vi "Enque Block (SubVI).vi"(10 "Block Parameters":T1={"Pixels In"=0, "BBox Array"=[0, 0, 0, 0, 0, 0, 0, 0, 0, 0, 0, 0, 0, 0, 0, 0], "Image Height"=0, "Image Width"=0, "Input Valid?"=FALSE, "Pixel Bus"={"Pixel Valid"=FALSE, "EOL"=FALSE, "EOF"=FALSE, "X"=0, "Y"=0}}, 11 "BOX ID":i32) -> (1 "Pixel Valid?":bool, 3 "Pixel Data":u8)   [LabVIEW 2015]
uses:
  Controls (FPGA)/Block Parameters.ctl
  Common/SubVIs (FPGA)/Pixel Bus.ctl
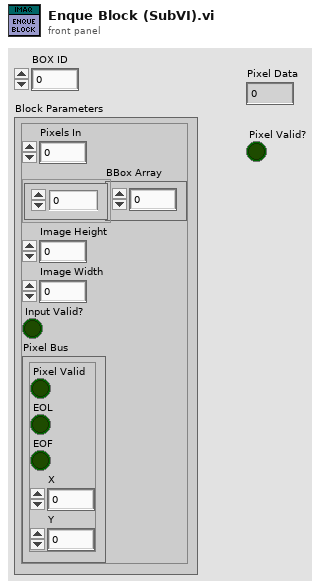
[diagram p1: front panel]
types:
  T1 = typedef "Block Parameters.ctl" = cluster{"Pixels In":u64, "BBox Array":u64[], "Image Height":u16, "Image Width":u16, "Input Valid?":bool, "Pixel Bus":T2}
  T2 = typedef "Pixel Bus.ctl" = cluster{"Pixel Valid":bool, "EOL":bool, "EOF":bool, "X":u16, "Y":u16}
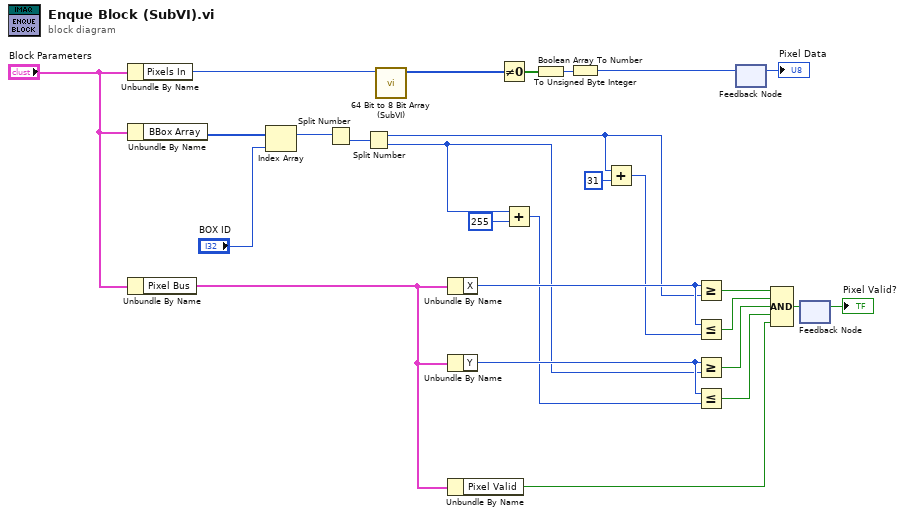
[diagram p0: block diagram]
diagram:
  n1 = Unbundle By Name("Block Parameters") -> ("Pixels In"=w24:u64)
  n2 = Unbundle By Name("Block Parameters") -> ("BBox Array"=w25:u64[])
  n3 = Unbundle By Name("Block Parameters") -> ("Pixel Bus"=w9:T2)
  n4 = Index Array(array=w25, index="BOX ID") -> (element=w23:u64)
  n5 = Split Number(x=w23) -> (lo(x)=w3:u32)  [unwired: 1 out]
  n6 = Split Number(x=w3) -> (hi(x)=w5:u16, lo(x)=w4:u16)
  n7 = call "64 Bit to 8 Bit Array (SubVI).vi"("Pixel In"=w24) -> ("Pixel Array Out"=w16:u8[])  [unwired: 10 in]
  n8 = Unbundle By Name(w9) -> ("X"=w12:u16)
  n9 = Unbundle By Name(w9) -> ("Y"=w11:u16)
  n10 = Unbundle By Name(w9) -> ("Pixel Valid"=w8:bool)
  n11 = Not Equal To 0?(x=w16) -> (x != 0?=w15:bool[])
  n12 = Add(x=w4, y=u16 255) -> (x+y=w6:u16)
  n13 = Boolean Array To Number(Boolean array=w15) -> (number=w14:u8)
  n14 = To Unsigned Byte Integer(number=w14) -> (unsigned 8bit integer=w13:u8)
  n15 = Add(x=w5, y=u16 31) -> (x+y=w7:u16)
  n16 = Greater Or Equal?(x=w12, y=w5) -> (x >= y?=w22:bool)
  n17 = Less Or Equal?(x=w12, y=w7) -> (x <= y?=w21:bool)
  n18 = Greater Or Equal?(x=w11, y=w4) -> (x >= y?=w20:bool)
  n19 = Less Or Equal?(x=w11, y=w6) -> (x <= y?=w19:bool)
  n20 = feedback #1() -> (→"Pixel Data":u8)  [unwired: 1 in]
  n21 = feedback-in #1(w13) -> ()
  n22 = Compound Arithmetic op=AND(w22, w21, w20, w19, w8) -> (w18:bool)
  n23 = feedback #2() -> (→"Pixel Valid?":bool)  [unwired: 1 in]
  n24 = feedback-in #2(w18) -> ()
